vi "Fusion Wavelets (with Measurements).vi"(6 "Fusion Method":cluster{"approximation":u16, "detail":u16}={"approximation"=2, "detail"=2} {"detail" items=["Max", "Min", "Mean", "Image 1", "Image 2"]; "approximation" items=["Max", "Min", "Mean", "Image 1", "Image 2"]}) -> ()   [LabVIEW 2023]
doc: "Computes the detail and approximation coefficients of two images using the WA Discrete Wavelet Transform VI, merges the resulting coefficients, and computes the fusion image using the WA Inverse Discrete Wavelet Transform VI."
uses:
  Images/_Images.ctl
panel:
  out "CNR":string[][](table)
  out "Image 2 (High Energy)":T1(plugin-control)
  out "Image 1 (Low energy)":T1(plugin-control)
  in  "Wavelet":u16(ring) items=["db02"=0, "db03"=1, "db04"=2, "db05"=3, "db06"=4, "db07"=5, "db08"=6, "db09"=7, "db10"=8, "db11"=9, "db12"=10, "db13"=11, "db14"=12, "Haar"=13, "bior1_3"=14, "bior1_5"=15, "bior2_2"=16, "bior2_4"=17, "bior2_6"=18, "bior2_8"=19, "bior3_1"=20, "bior3_3"=21, "bior3_5"=22, "bior3_7"=23, "bior3_9"=24, "bior4_4 (FBI)"=25, "bior5_5"=38, "bior6_8"=39, "coif1"=26, "coif2"=27, "coif3"=28, "coif4"=29, "coif5"=30, "sym2"=31, "sym3"=32, "sym4"=33, "sym5"=34, "sym6"=35, "sym7"=36, "sym8"=37]
  out "Fusion":T1(plugin-control)
  # "Images Fusion using Wavelets"
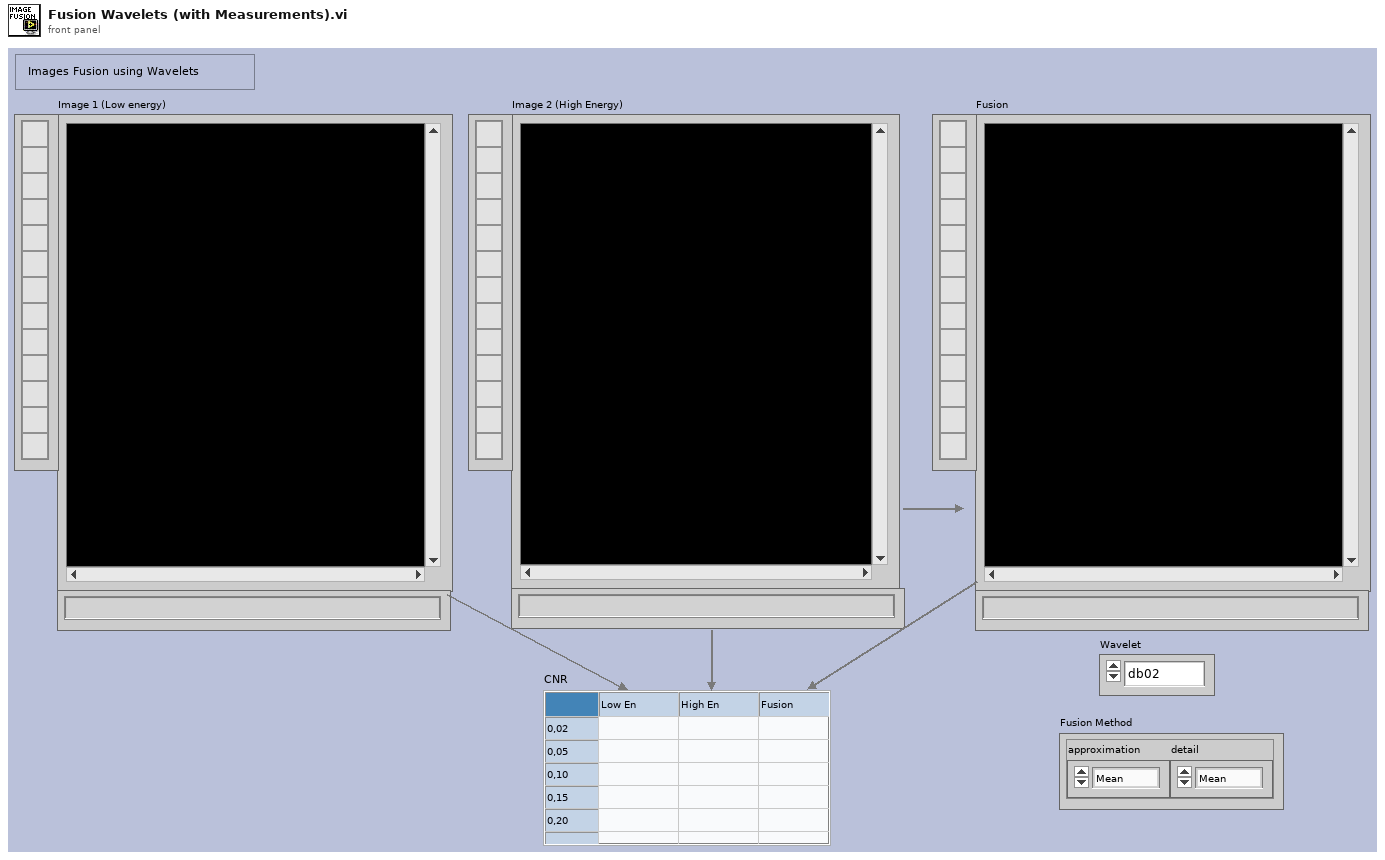
[diagram p1: front panel]
types:
  T1 = typedef "IMAQ Image.ctl" = refnum<image>
  T2 = typedef "IMAQ Point" = cluster{"X":sgl, "Y":sgl}
  T3 = typedef "Image Type" = u32
  T4 = typedef "_Images.ctl" = enum16{"Balls2", "Battery1", "Battery2", "Connector1", "Subwoofer1", "Subwoofer2", "Subwoofer3", "Subwoofer4", "Hase1", "Lamp1", "Lamp2", "Mouse1", "PhotoLens1", "Po1", "PowerSupply1", "Router", "--- Step Wedges ---", "Stepwedge1", "Stepwedge2", "Stepwedge3", "--- Fusion ---", "Fusion160kV", "Fusion2-120kV", "Fusion2-320kV", "Fusion300kV", "FusionPart1-120kV", "FusionPart1-180kV", "--- PART 01 ---", "Part1", "Part2", "Part3", "Part4", "Part5", "Part6", "Part7", "Part8", "--- Different Integrations ---", "Step2737-02Int", "Step2737-04Int", "Step2737-08Int", "Step2737-16Int", "Step2737-32Int", "Step2737-64Int"}
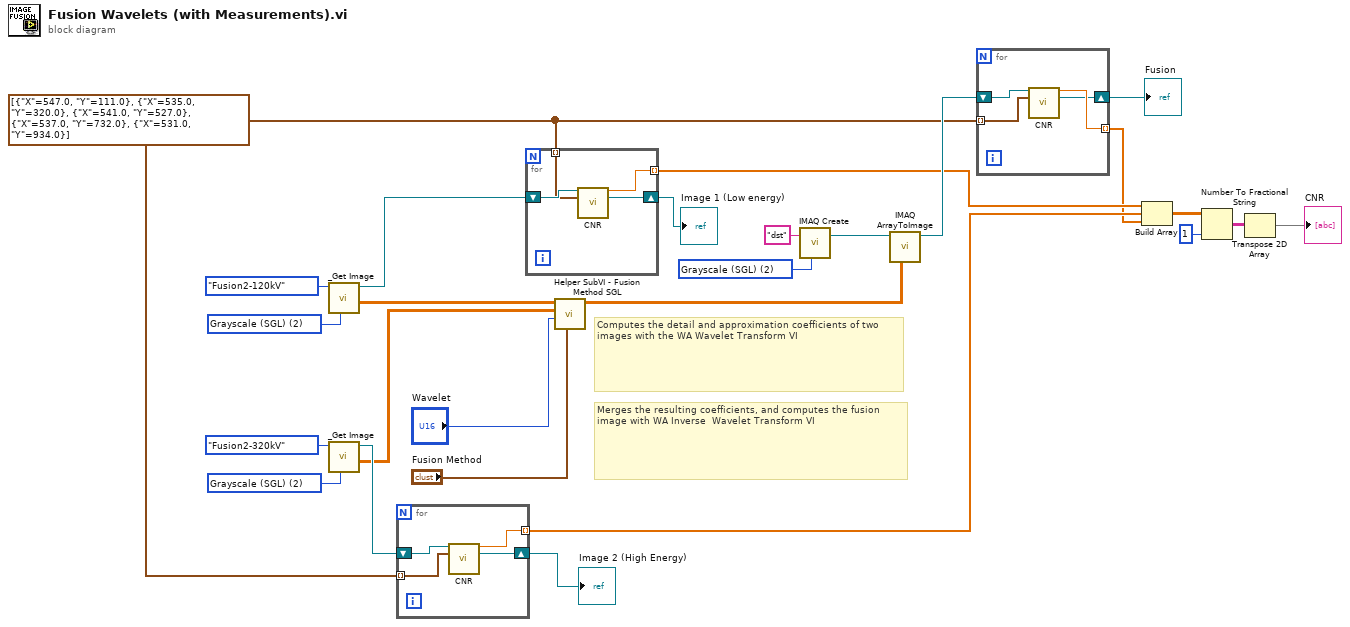
[diagram p0: block diagram]
diagram:
  w13 = T2[] [{"X"=547.0, "Y"=111.0}, {"X"=535.0, "Y"=320.0}, {"X"=541.0, "Y"=527.0}, {"X"=537.0, "Y"=732.0}, {"X"=531.0, "Y"=934.0}]
  w19 = T3 2 items=["Grayscale (U8)", "Grayscale (I16)", "Grayscale (SGL)", "Complex (CSG)", "RGB (U32)", "HSL (U32)", "RGB (U64)", "Grayscale (U16)"] ("Image Type (U16)")
  w21 = T3 2 items=["Grayscale (U8)", "Grayscale (I16)", "Grayscale (SGL)", "Complex (CSG)", "RGB (U32)", "HSL (U32)", "RGB (U64)", "Grayscale (U16)"] ("Image Type")
  w23 = T3 2 items=["Grayscale (U8)", "Grayscale (I16)", "Grayscale (SGL)", "Complex (CSG)", "RGB (U32)", "HSL (U32)", "RGB (U64)", "Grayscale (U16)"] ("Image Type (U16)")
  # "Merges the resulting coefficients, and computes the fusion image with WA Inverse  Wavelet Transform VI"
  # "Computes the detail and approximation coefficients of two images with the WA Wavelet Transform VI"
  n1 = call "_Get Image.vi"("Image Type (U16)"=w23, "Image"=_Images."Fusion2-120kV") -> ("Image Pixels (Float)"=w3:dbl[][], "Image Out"=w15:T1)  [unwired: 6 in, 2 out]
  n2 = call "_Get Image.vi"("Image Type (U16)"=w19, "Image"=_Images."Fusion2-320kV") -> ("Image Pixels (Float)"=w2:dbl[][], "Image Out"=w12:T1)  [unwired: 6 in, 2 out]
  n3 = for {
    tunnel: w13 -> [w29] mode=indexing
    shift-right: [w27] -> w11
    shift-left: w12 -> [w30]
    tunnel: [w28] -> w9 mode=indexing
    n4 = call "CNR.vi"("Image In"=w30, "Point"=w29) -> ("CNR"=w28:dbl, "Image"=w27:T1)  [unwired: 8 in, 4 out]
  }
  "Image 2 (High Energy)" <- w11
  n5 = for {
    tunnel: w13 -> [w33] mode=indexing
    shift-right: [w31] -> w14
    shift-left: w15 -> [w34]
    tunnel: [w32] -> w10 mode=indexing
    n6 = call "CNR.vi"("Image In"=w34, "Point"=w33) -> ("CNR"=w32:dbl, "Image"=w31:T1)  [unwired: 8 in, 4 out]
  }
  "Image 1 (Low energy)" <- w14
  n7 = call "Helper SubVI - Fusion Method SGL.vi"("Fusion Method"="Fusion Method", "Wavelet"="Wavelet", "Image Pixels (Float)"=w2, "Image Pixels (Float) 2"=w3) -> ("Array"=w18:sgl[][])  [unwired: 7 in]
  n8 = call "IMAQ Create"("Image Name"="dst", "Image Type"=w21) -> ("New Image"=w20:T1)  [unwired: 3 in, 1 out]
  n9 = call "IMAQ ArrayToImage"("Image Pixels (Float)"=w18, "Image"=w20) -> ("Image Out"=w17:T1)  [unwired: 8 in, 1 out]
  n10 = for {
    tunnel: w13 -> [w37] mode=indexing
    shift-right: [w35] -> w16
    shift-left: w17 -> [w38]
    tunnel: [w36] -> w8 mode=indexing
    n11 = call "CNR.vi"("Image In"=w38, "Point"=w37) -> ("CNR"=w36:dbl, "Image"=w35:T1)  [unwired: 8 in, 4 out]
  }
  "Fusion" <- w16
  n12 = Build Array(w10, w9, w8) -> (w7:dbl[][])
  n13 = Number To Fractional String(number=w7, precision (6)=i16 1) -> (F-format string=w6:string[][])  [unwired: 2 in]
  n14 = Transpose 2D Array(2D array=w6) -> (transposed array=→"CNR":string[][])
